vi "CODMn启动命令 (子VI).vi"(9 "强制切换":bool, 10 "CODMn量程切换":enum32{"H", "L", "AUTO"}(ring)=enum."AUTO", 11 "启动测量模式":T1) -> ()   [LabVIEW 2016, in "斯坦道CODMn.lvlib"]
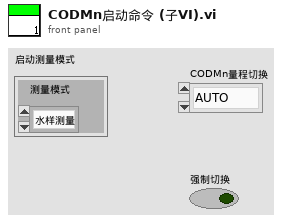
[diagram p1: front panel]
types:
  T1 = cluster{"测量模式":enum16{"水样测量", "标样核查", "零点核查", "跨度核查", "空白测试", "加标回收", "平行样", "校零", "校标"}}
  T2 = enum16{"水样测量", "标样核查", "零点核查", "跨度核查", "空白测试", "加标回收", "平行样", "校零", "校标"}
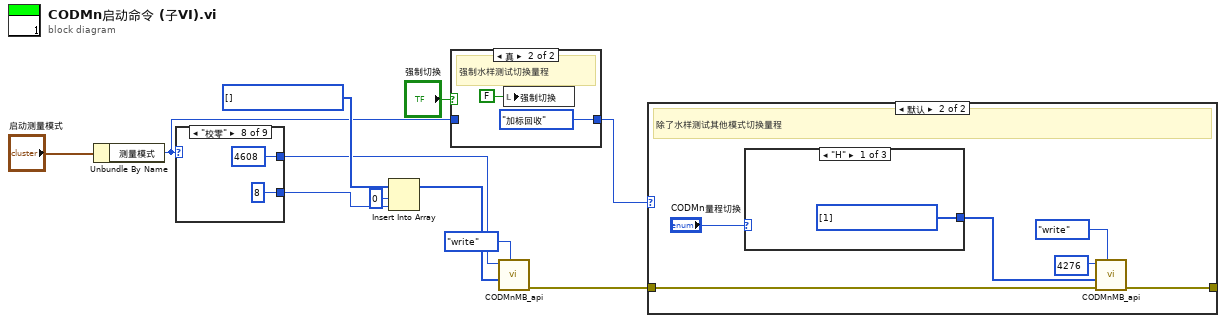
[diagram p0: block diagram]
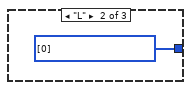
[diagram p4: hidden frame]
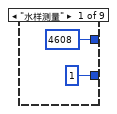
[diagram p6: hidden frame]
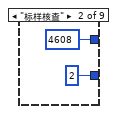
[diagram p7: hidden frame]
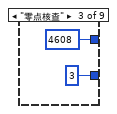
[diagram p8: hidden frame]
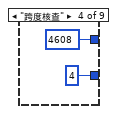
[diagram p9: hidden frame]
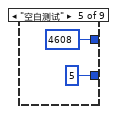
[diagram p10: hidden frame]
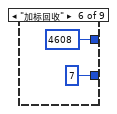
[diagram p11: hidden frame]
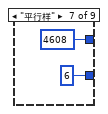
[diagram p12: hidden frame]
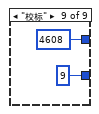
[diagram p13: hidden frame]
diagram:
  n1 = Unbundle By Name("启动测量模式") -> ("测量模式"=w7:T2)
  n2 = case shown="\"校零\"" w7 {
    tunnel: [u16 4608 ("address") u16 4608 ("address") u16 4608 ("address") u16 4608 ("address") u16 4608 ("address") u16 4608 ("address") u16 4608 ("address") u16 4608 ("address") u16 4608 ("address")] -> w2
    tunnel: [u16 1 ("address") u16 2 ("address") u16 3 ("address") u16 4 ("address") u16 5 ("address") u16 7 ("address") u16 6 ("address") u16 8 ("address") u16 9 ("address")] -> w10
    frame "水样测量" {
    }
    frame "标样核查" {
    }
    frame "零点核查" {
    }
    frame "跨度核查" {
    }
    frame "空白测试" {
    }
    frame "加标回收" {
    }
    frame "平行样" {
    }
    frame "校零" {
    }
    frame "校标" {
    }
  }
  n3 = Insert Into Array(array=u16[] [] ("values"), index=0 ("索引"), new element=w10) -> (w1:u16[])
  n4 = case shown="真" "强制切换" {
    tunnel: w7 -> [w30 _]
    tunnel: [w30 T2."加标回收" ("测量模式")] -> w6
    frame False {
    }
    frame True {
      # "强制水样测试切换量程"
      n5 = local write "强制切换"(FALSE ("强制切换")) -> ()
    }
  }
  n6 = call "CODMnMB_api.vi"("STEP"=enum16{"open", "read", "write", "close"}."write", "values"=w1, "starting address"=w2) -> ("error out"=w3:errorcluster)  [unwired: 6 in, 2 out]
  n7 = case shown="默认" w6 {
    tunnel: w3 -> [w33 w35]
    tunnel: [w33 w34] -> _
    frame "水样测量" {
      # "水样测试不切换"
    }
    frame Default {
      # "除了水样测试其他模式切换量程"
      n8 = case shown="\"H\"" "CODMn量程切换" {
        tunnel: [u16[] [1] ("values") u16[] [0] ("values") _] -> w36
        frame "H" {
        }
        frame "L" {
        }
        frame "AUTO", Default {
        }
      }
      n9 = call "CODMnMB_api.vi"("STEP"=enum16{"open", "read", "write", "close"}."write", "Error in"=w35, "values"=w36, "starting address"=u16 4276) -> ("error out"=w34:errorcluster)  [unwired: 5 in, 2 out]
    }
  }
